vi "CMN_toUnsc.vi"(3 "responseQ":string, 4 "ms timeout (-1)":i32=-1, 5 "key":string, 6 "bpp":i32, 7 "location 2":u64, 8 "error in (no error)":errorcluster, 9 "ele Read":u32, 10 "location":u64, 11 "command":string) -> (0 "error out":errorcluster, 1 "response":errorcluster)   [LabVIEW 2016]
panel:
  in  "command strct":T1
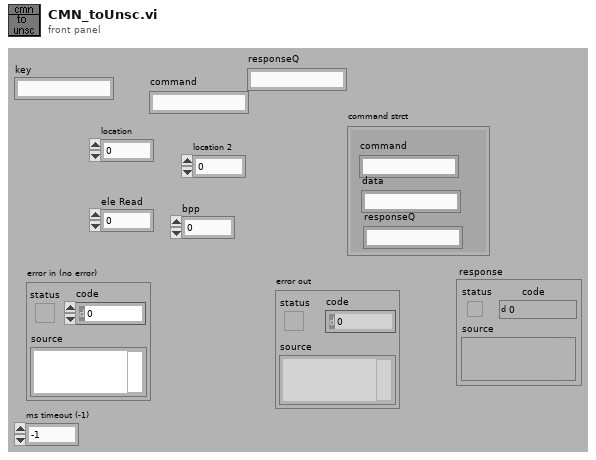
[diagram p1: front panel]
types:
  T1 = cluster{"command":string, "data":string, "responseQ":string}
  T2 = cluster{"location":u64, "ele Read":u32, "location 2":u64, "bpp":i32}
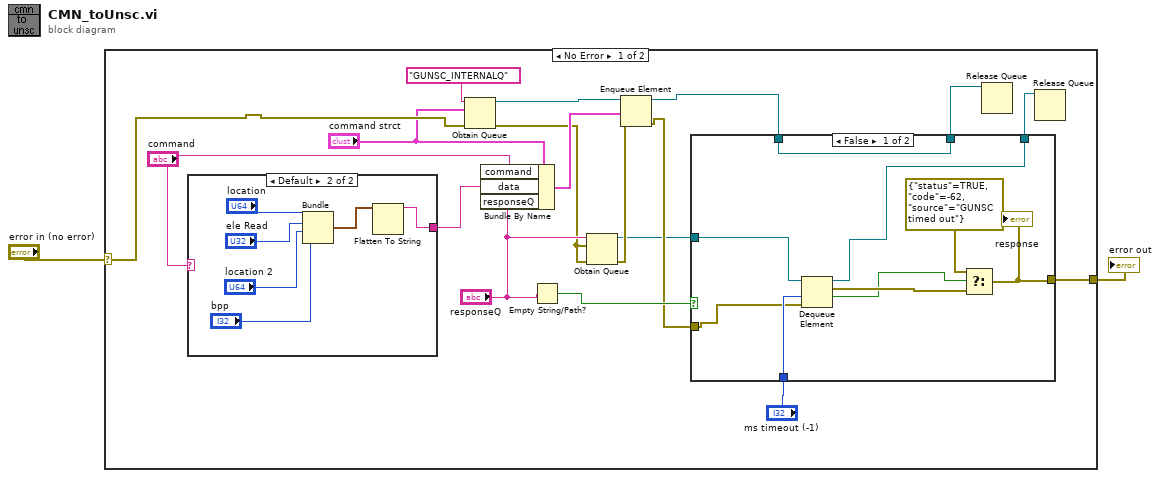
[diagram p0: block diagram]
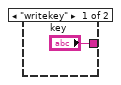
[diagram p3: hidden frame]
diagram:
  n1 = case shown="No Error" "error in (no error)" {
    selector: "error in (no error)" -> [w14 w40]
    tunnel: [w16 w40] -> w1
    frame No Error {
      n2 = case shown="Default" "command" {
        tunnel: ["key" w36] -> w20
        frame "writekey" {
        }
        frame Default {
          n3 = Bundle("location"="location", "ele Read"="ele Read", "location 2"="location 2", "bpp"="bpp") -> (w37:T2)  [unwired: 1 out]
          n4 = Flatten To String(anything=w37) -> (data string=w36:string)  [unwired: 1 in, 4 out]
        }
      }
      n5 = Obtain Queue(name (unnamed)="GUNSC_INTERNALQ", element data type="command strct", error in (no error)=w14) -> (queue out=w11:refnum<queue>, error out=w3:errorcluster)  [unwired: 2 in, 1 out]
      n6 = Bundle By Name(cluster="command strct", "command"="command", "data"=w20, "responseQ"="responseQ") -> (w10:T1)
      n7 = Empty String/Path?(string/path="responseQ") -> (empty?=w18:bool)
      n8 = Obtain Queue(name (unnamed)="responseQ", element data type=w3, error in (no error)=w3) -> (queue out=w5:refnum<queue>, error out=w6:errorcluster)  [unwired: 2 in, 1 out]
      n9 = Enqueue Element(queue=w11, element=w10, error in (no error)=w6) -> (queue out=w9:refnum<queue>, error out=w12:errorcluster)  [unwired: 2 out]
      n10 = case shown="False" w18 {
        tunnel: "ms timeout (-1)" -> [w27 _]
        tunnel: w12 -> [w21 w32]
        tunnel: [w28 w32] -> w16
        tunnel: w9 -> [w24 w31]
        tunnel: [w24 w31] -> w8
        tunnel: [w23 w30] -> w7
        tunnel: w5 -> [w22 w30]
        frame False {
          n11 = Dequeue Element(queue=w22, timeout in ms (-1)=w27, error in (no error)=w21) -> (queue out=w23:refnum<queue>, element=w26:errorcluster, timed out?=w25:bool)  [unwired: 1 out]
          n12 = Select(t=errorcluster {"status"=TRUE, "code"=-62, "source"="GUNSC timed out"}, s=w25, f=w26) -> (s? t:f=w28:errorcluster)
          "response" <- w28
        }
        frame True {
        }
      }
      n13 = Release Queue(queue=w8) -> ()  [unwired: 1 in, 4 out]
      n14 = Release Queue(queue=w7) -> ()  [unwired: 1 in, 4 out]
    }
    frame Error {
    }
  }
  "error out" <- w1
